vi "Read Serial data array.vi"(8 "error in (no error)":errorcluster, 11 "Serial Array in":refnum<visa-resource-name>[](array[refnum])) -> (0 "error out":errorcluster, 1 "Serial cluster array":T1[](array[typedef]), 2 "Buffer array":string[](array[string]), 3 "Serial Array out":refnum<visa-resource-name>[](array[refnum]), 5 "Trip pressure array":dbl[](array[numeric]))   [LabVIEW 2019]
uses:
  sandbox/Instrument.AML.GetAll--Cluster.ctl
  Program Files (x86)/National Instruments/LabVIEW 2019/examples/Instrument IO/Serial/support/Serial - Settings.ctl
  <vilib>/Instr/_visa.llb/VISA Configure Serial Port (Instr).vi
panel:
  out "read buffer":string
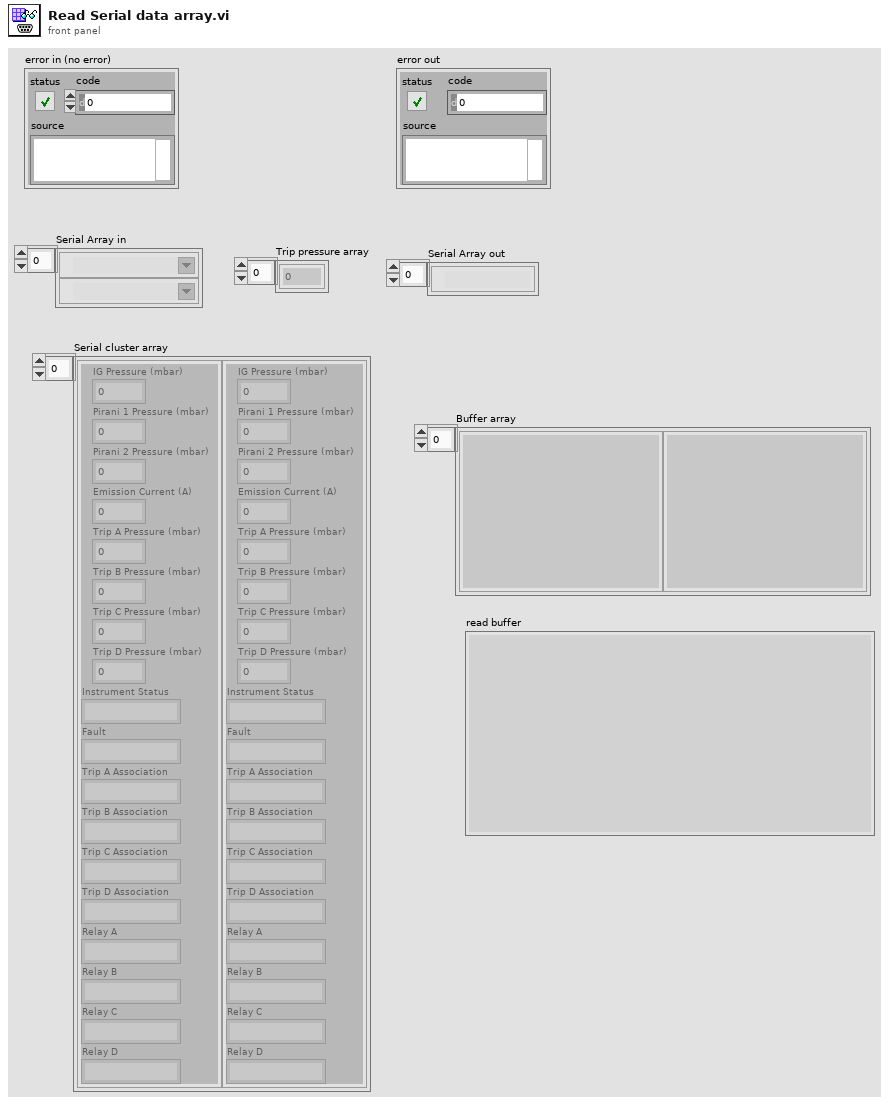
[diagram p1: front panel]
types:
  T1 = typedef "Instrument.AML.GetAll--Cluster.ctl" = cluster{"IG Pressure (mbar)":dbl, "Pirani 1 Pressure (mbar)":dbl, "Pirani 2 Pressure (mbar)":dbl, "Emission Current (A)":dbl, "Trip A Pressure (mbar)":dbl, "Trip B Pressure (mbar)":dbl, "Trip C Pressure (mbar)":dbl, "Trip D Pressure (mbar)":dbl, "Instrument Status":string, "Fault":string, "Trip A Association":string, "Trip B Association":string, "Trip C Association":string, "Trip D Association":string, "Relay A":string, "Relay B":string, "Relay C":string, "Relay D":string}
  T2 = typedef "Serial - Settings.ctl" = cluster{"baud rate":u32, "data bits":u16, "parity":enum16{"None", "Odd", "Even", "Mark", "Space"}, "stop bits":u16, "flow control":u16}
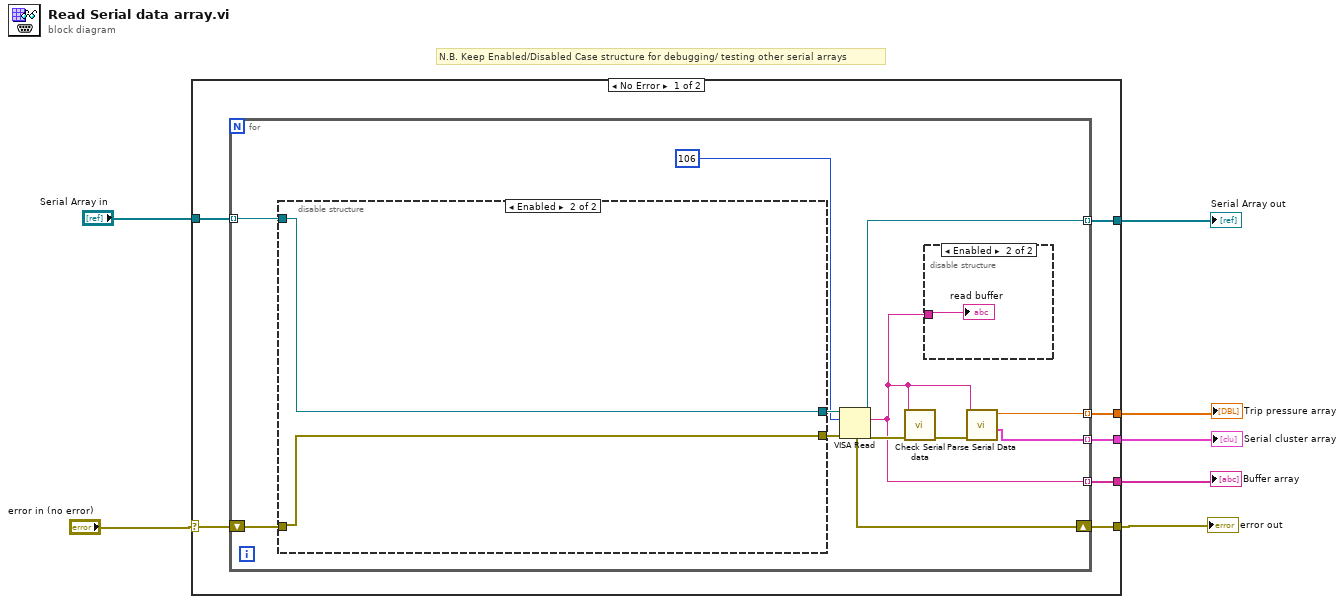
[diagram p0: block diagram]
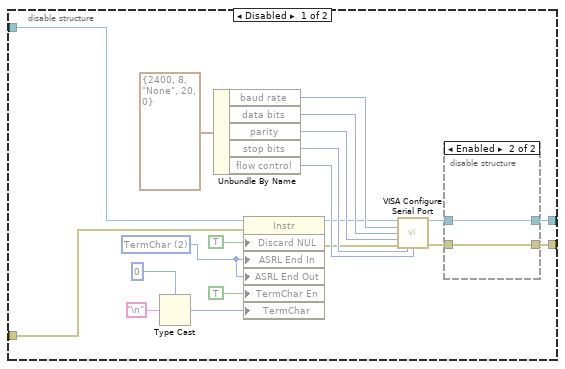
[diagram p2: hidden frame]
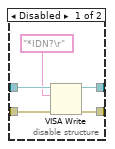
[diagram p3: hidden frame]
diagram:
  # "N.B. Keep Enabled/Disabled Case structure for debugging/ testing other serial arrays"
  n1 = case shown="No Error" "error in (no error)" {
    selector: "error in (no error)" -> [w13 w58]
    tunnel: [w14 w58] -> w7
    tunnel: [w12 w57] -> w3
    tunnel: "Serial Array in" -> [w11 w57]
    tunnel: [w10 _] -> w6
    tunnel: [w9 _] -> w5
    tunnel: [w8 _] -> w4
    frame No Error {
      n2 = for {
        tunnel: [w15] -> w10 mode=indexing
        shift-right: [w23] -> w14
        shift-left: w13 -> [w17]
        tunnel: [w26] -> w12 mode=indexing
        tunnel: w11 -> [w20] mode=indexing
        tunnel: [w22] -> w9 mode=indexing
        tunnel: [w21] -> w8 mode=indexing
        n3 = disable-structure shown="Enabled" {
          disable-tunnel: w20 -> [w30 w55]
          disable-tunnel: [w29 w55] -> w19
          disable-tunnel: [w28 w54] -> w18
          disable-tunnel: w17 -> [w27 w54]
          frame Disabled {
            w41 = u16 2 items=["None", "Last Bit", "TermChar"] ("Serial Settings:End Mode for Reads")
            n4 = Type Cast(type=0, x="\n") -> (*(type *) &x=w38:i32)
            n5 = Unbundle By Name(T2 {"baud rate"=2400, "data bits"=8, "parity"=enum."None", "stop bits"=20, "flow control"=0} ("input cluster")) -> ("baud rate"=w46:u32, "data bits"=w45:u16, "parity"=w44:enum16{"None", "Odd", "Even", "Mark", "Space"}, "stop bits"=w43:u16, "flow control"=w42:u16)
            n6 = property class="Instr"(reference=w30, error in=w27, "Discard NUL"=TRUE ("Serial Settings:Discard NUL Characters"), "ASRL End In"=w41, "ASRL End Out"=w41, "TermChar En"=TRUE ("Message Based Settings:Termination Character Enable"), "TermChar"=w38) -> (reference out=w36:refnum<visa-resource-name>, error out=w37:errorcluster)
            n7 = call-poly "VISA Configure Serial Port"("VISA resource name"=w36, "baud rate (9600)"=w46, "data bits (8)"=w45, "parity (0:none)"=w44, "error in (no error)"=w37, "stop bits (10: 1 bit)"=w43, "flow control (0:none)"=w42) -> ("VISA resource name out"=w32:refnum<visa-resource-name>, "error out"=w35:errorcluster)  [unwired: 7 in]
            n8 = disable-structure shown="Enabled" {
              disable-tunnel: w35 -> [w51 w52]
              disable-tunnel: w32 -> [w50 w53]
              disable-tunnel: [w48 w53] -> w29
              disable-tunnel: [w47 w52] -> w28
              frame Disabled {
                n9 = VISA Write(VISA resource name=w50, write buffer="*IDN?\r" ("Command"), error in (no error)=w51) -> (VISA resource name out=w48:refnum<visa-resource-name>, error out=w47:errorcluster)  [unwired: 1 out]
              }
              frame Enabled {
              }
            }
          }
          frame Enabled {
          }
        }
        n10 = VISA Read(VISA resource name=w19, byte count=u32 106, error in (no error)=w18) -> (VISA resource name out=w26:refnum<visa-resource-name>, read buffer=w15:string, error out=w25:errorcluster)  [unwired: 1 out]
        n11 = call "Check Serial data.vi"("error in"=w25, "Buffer in"=w15) -> ("error IO"=w24:errorcluster)  [unwired: 8 in, 1 out]
        n12 = disable-structure shown="Enabled" {
          disable-tunnel: w15 -> [_ w56]
          frame Disabled {
          }
          frame Enabled {
            "read buffer" <- w56
          }
        }
        n13 = call "Parse Serial Data.vi"("error in"=w24, "Buffer in"=w15) -> ("error IO"=w23:errorcluster, "cluster"=w22:T1, "Trip pressure"=w21:dbl)  [unwired: 7 in]
      }
    }
    frame Error {
    }
  }
  "Serial Array out" <- w3
  "Trip pressure array" <- w4
  "Serial cluster array" <- w5
  "Buffer array" <- w6
  "error out" <- w7
